vi "Define one period (SubVI).vi"(9 "Index":dbl, 10 "Array in":dbl[](array[numeric])) -> (0 "element":dbl, 3 "One period?":bool)   [LabVIEW 2018]
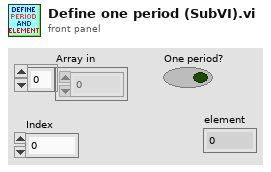
[diagram p1: front panel]
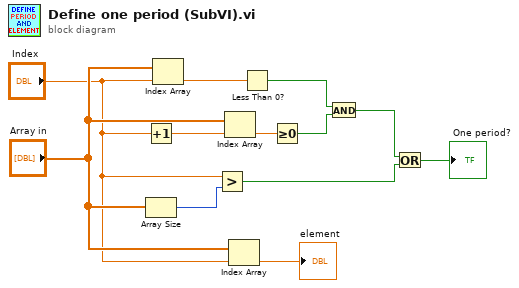
[diagram p0: block diagram]
diagram:
  n1 = Increment(x="Index") -> (x+1=w8:dbl)
  n2 = Array Size(array="Array in") -> (size(s)=w7:i32)
  n3 = Index Array(array="Array in", index="Index") -> (element=w9:dbl)
  n4 = Greater?(x="Index", y=w7) -> (0:w6:bool)
  n5 = Index Array(array="Array in", index=w8) -> (element=w12:dbl)
  n6 = Index Array(array="Array in", index="Index") -> (element=→"element":dbl)
  n7 = Less Than 0?(x=w9) -> (x < 0?=w10:bool)
  n8 = Greater Or Equal To 0?(x=w12) -> (x >= 0?=w11:bool)
  n9 = And(x=w10, y=w11) -> (x .and. y?=w5:bool)
  n10 = Or(x=w5, y=w6) -> (x .or. y?=→"One period?":bool)
